vi "SetFreqOffset_Addon.vi"(6 "Resp Timeout (ms)":i32 min=0, 7 "Enum":T1, 8 "Error In":errorcluster, 10 "Freq Offset (Hz)":i64=1, 11 "FPGA Reference":refnum<k20>) -> (0 "Error Out":errorcluster, 1 "Received Text":string, 2 "Set Freq Offset OK":bool, 3 "Sent Text":string)   [LabVIEW 2018]
uses:
  Resources_Test/UART/ControlTestSlot.ctl
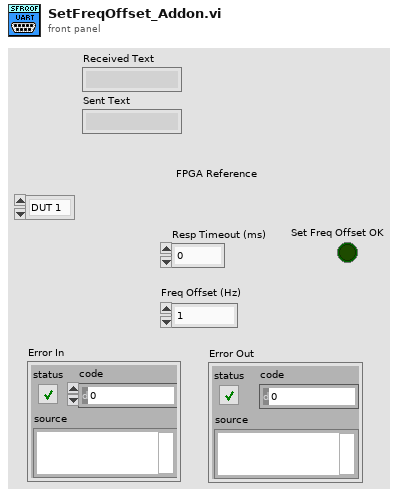
[diagram p1: front panel]
types:
  T1 = typedef "ControlTestSlot.ctl" = enum16{"DUT 1", "DUT 2"}
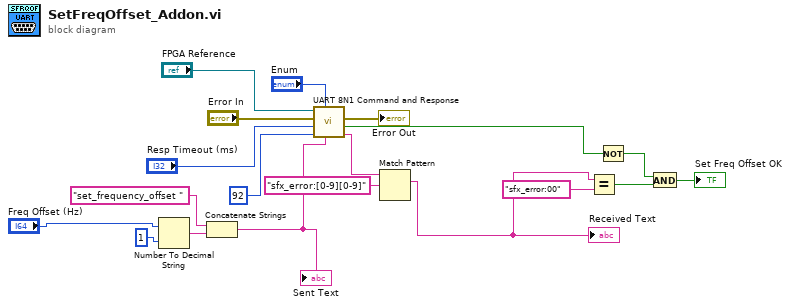
[diagram p0: block diagram]
diagram:
  n1 = Number To Decimal String(number="Freq Offset (Hz)", width (-)=i16 1) -> (decimal integer string=w14:string)
  n2 = Concatenate Strings("set_frequency_offset " ("Text to Send"), w14) -> (w8:string)
  "Sent Text" <- w8
  n3 = call "UART 8N1 Command and Response.vi"("Text to Send"=w8, "Active Dut"="Enum", "Response Size (char)"=u32 92, "Response Timeout (ms)"="Resp Timeout (ms)", "Error In"="Error In", "FPGA VI Reference In"="FPGA Reference") -> ("Received Text"=w3:string, "Timeout Flag"=w6:bool, "Error Out"=→"Error Out":errorcluster)  [unwired: 1 in, 2 out]
  n4 = Match Pattern(string=w3, regular expression="sfx_error:[0-9][0-9]") -> (match substring=w1:string)  [unwired: 1 in, 3 out]
  "Received Text" <- w1
  n5 = Equal?(x=w1, y="sfx_error:00") -> (x = y?=w17:bool)
  n6 = Not(x=w6) -> (.not. x?=w19:bool)
  n7 = And(x=w19, y=w17) -> (x .and. y?=→"Set Freq Offset OK":bool)
